vi "obtain_linked_point.vi"(8 "error in (no error)":errorcluster, 10 "point ID":dbl, 11 "PointLinkCollection in":refnum<class "PointLinkCollection.lvclass">) -> (0 "error out":errorcluster, 1 "found?":bool, 2 "linked point ID":dbl, 3 "PointLinkCollection out":refnum<class "PointLinkCollection.lvclass">)   [LabVIEW 2010, in "PointLinkCollection.lvclass"]
uses:
  PointLinkCollection.lvclass
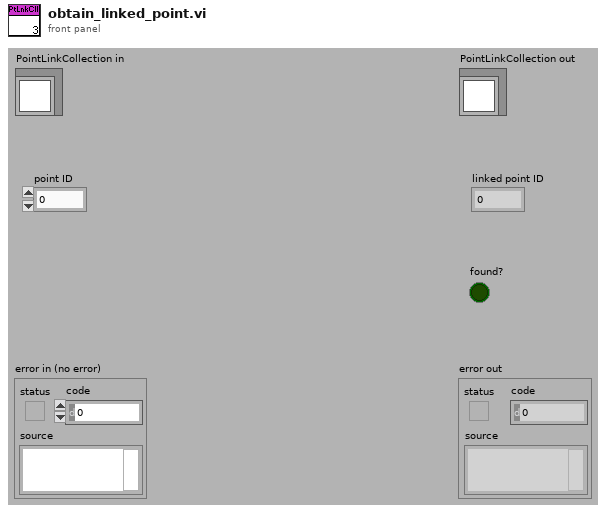
[diagram p1: front panel]
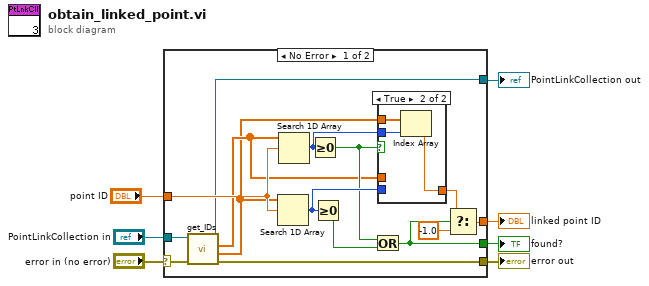
[diagram p0: block diagram]
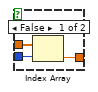
[diagram p2: hidden frame]
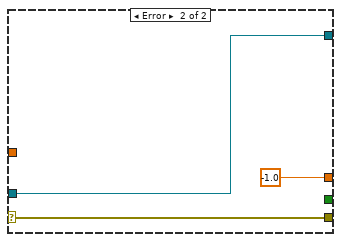
[diagram p3: hidden frame]
diagram:
  n1 = case shown="No Error" "error in (no error)" {
    selector: "error in (no error)" -> [w9 w31]
    tunnel: [w8 w31] -> w6
    tunnel: [w10 w30] -> w4
    tunnel: "PointLinkCollection in" -> [w11 w30]
    tunnel: "point ID" -> [w22 _]
    tunnel: [w15 -1.0 ("f")] -> w2
    tunnel: [w17 _] -> w1
    frame No Error {
      n2 = call "get_IDs.vi"("error in (no error)"=w9, "PointLinkCollection in"=w11) -> ("error out"=w8:errorcluster, "IDs B"=w12:dbl[], "IDs A"=w13:dbl[], "PointLinkCollection out"=w10:refnum<class "PointLinkCollection.lvclass">)  [unwired: 5 in, 1 out]
      n3 = Search 1D Array(1D array=w12, element=w22) -> (index of element=w20:i32)  [unwired: 1 in]
      n4 = Search 1D Array(1D array=w13, element=w22) -> (index of element=w21:i32)  [unwired: 1 in]
      n5 = Greater Or Equal To 0?(x=w21) -> (x >= 0?=w19:bool)
      n6 = Greater Or Equal To 0?(x=w20) -> (x >= 0?=w18:bool)
      n7 = Or(x=w19, y=w18) -> (x .or. y?=w17:bool)
      n8 = case shown="True" w19 {
        tunnel: w21 -> [_ w28]
        tunnel: w12 -> [_ w27]
        tunnel: w13 -> [w25 _]
        tunnel: w20 -> [w24 _]
        tunnel: [w23 w26] -> w14
        frame False {
          n9 = Index Array(array=w25, index=w24) -> (element=w23:dbl)
        }
        frame True {
          n10 = Index Array(array=w27, index=w28) -> (element=w26:dbl)
        }
      }
      n11 = Select(t=w14, s=w17, f=-1.0) -> (s? t:f=w15:dbl)
    }
    frame Error {
    }
  }
  "error out" <- w6
  "PointLinkCollection out" <- w4
  "linked point ID" <- w2
  "found?" <- w1
